vi "Recorder set.vi"(4 "Memory(0~9)":u32 max=9, 5 "Name":string, 6 "Set Memory or USB (T:USB F:Memory)":bool, 7 "Channel  (1: CH1)":u16(ring)=1 items=["CH1"=1, "CH2"=2, "CH3"=3, "CH4"=4], 8 "error in (no error)":errorcluster, 9 "Groups(1~2048)":u32=1 min=1 max=2048, 10 "Period(1s~300s)":u32=1 min=1 max=300, 11 "VISA resource name":refnum<visa-resource-name>) -> (0 "error out":errorcluster, 3 "VISA resource name out":refnum<visa-resource-name>)   [LabVIEW 2020, in "GPP.lvlib"]
uses:
  GPP.lvlib
  Function/VISA_COMMON.ctl
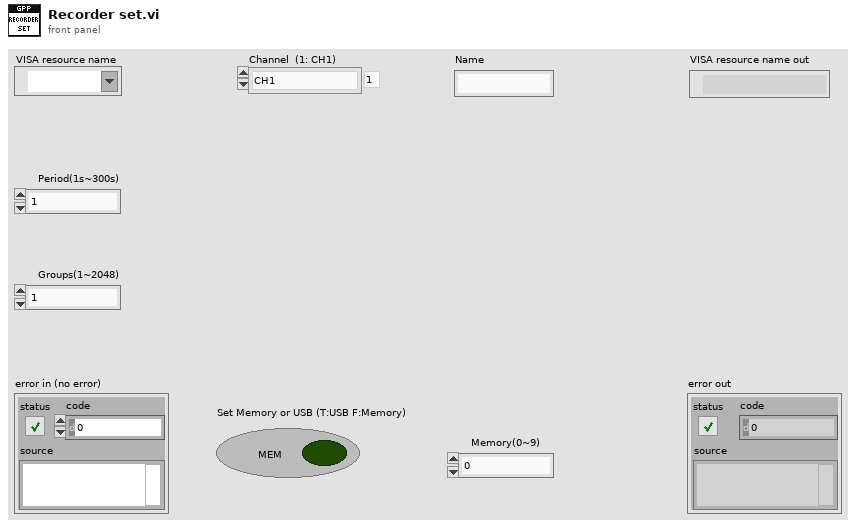
[diagram p1: front panel]
types:
  T1 = typedef "GPP.lvlib/VISA_COMMON.ctl" = enum16{"Initial", "Write CMD", "Read Result", "Read History", "Close"}
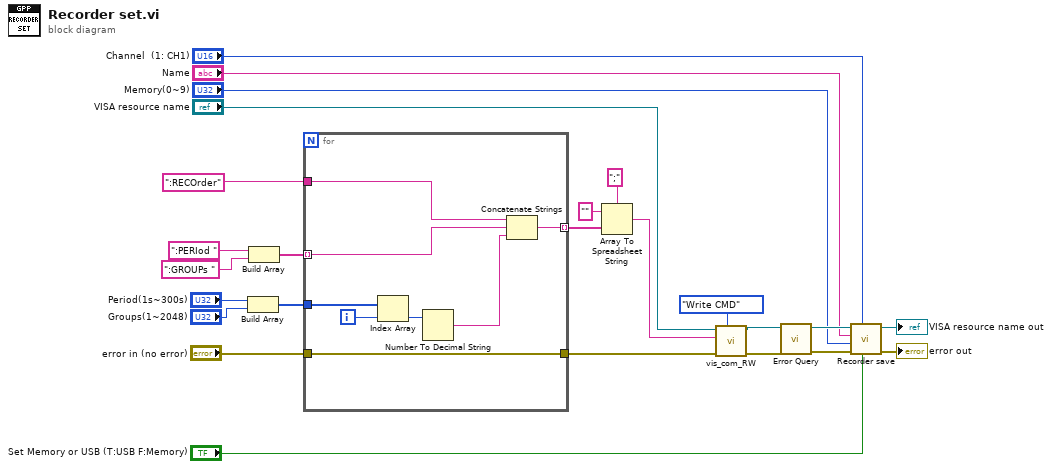
[diagram p0: block diagram]
diagram:
  n1 = Build Array("Period(1s~300s)", "Groups(1~2048)") -> (w11:u32[])
  n2 = Build Array(":PERIod ", ":GROUPs ") -> (w14:string[])
  n3 = for {
    tunnel: w14 -> [w32] mode=indexing
    tunnel: w11 -> [w29]
    tunnel: [w31] -> w18
    tunnel: "error in (no error)" -> [w31]
    tunnel: [w30] -> w16 mode=indexing
    tunnel: ":RECOrder" -> [w27]
    i -> [w28]
    n4 = Index Array(array=w29, index=w28) -> (element=w26:u32)
    n5 = Number To Decimal String(number=w26) -> (decimal integer string=w33:string)  [unwired: 1 in]
    n6 = Concatenate Strings(w27, w32, w33) -> (w30:string)
  }
  n7 = Array To Spreadsheet String(delimiter (Tab)=";", array=w16, 3:"" ("format string")) -> (spreadsheet string=w10:string)
  n8 = call "vis_com_RW.vi"("Funciton"=VISA_COMMON."Write CMD", "error in (no error)"=w18, "CMD String"=w10, "VISA resource in"="VISA resource name") -> ("error out"=w22:errorcluster, "VISA resource out"=w23:refnum<visa-resource-name>)  [unwired: 5 in, 1 out]
  n9 = call "Error Query.vi"("error in (no error)"=w22, "VISA resource name"=w23) -> ("error out"=w5:errorcluster, "VISA resource name out"=w8:refnum<visa-resource-name>)  [unwired: 6 in, 2 out]
  n10 = call "Recorder save.vi"("Set Memory or USB (T:USB F:Memory)"="Set Memory or USB (T:USB F:Memory)", "Channel  (1: CH1)"="Channel  (1: CH1)", "error in (no error)"=w5, "Memory(0~9)"="Memory(0~9)", "Name"="Name", "VISA resource name"=w8) -> ("error out"=→"error out":errorcluster, "VISA resource name out"=→"VISA resource name out":refnum<visa-resource-name>)  [unwired: 4 in]
